vi "LaserCalibration.vi"() -> ()   [LabVIEW 2012]
uses:
  <vilib>/Utility/file.llb/Read From Spreadsheet File (DBL).vi
  <vilib>/Utility/file.llb/Write To Spreadsheet File (DBL).vi
  <vilib>/Analysis/NI_AALPro.lvlib
panel:
  out "slope 2":dbl
  out "slope":dbl
  out "Power vs. Voltage":cluster{"all rows":dbl[], "all rows":dbl[]}[](graph)
  out "Output Voltage":dbl(knob) scale=0.0..5.0
  in  "Steps":i32
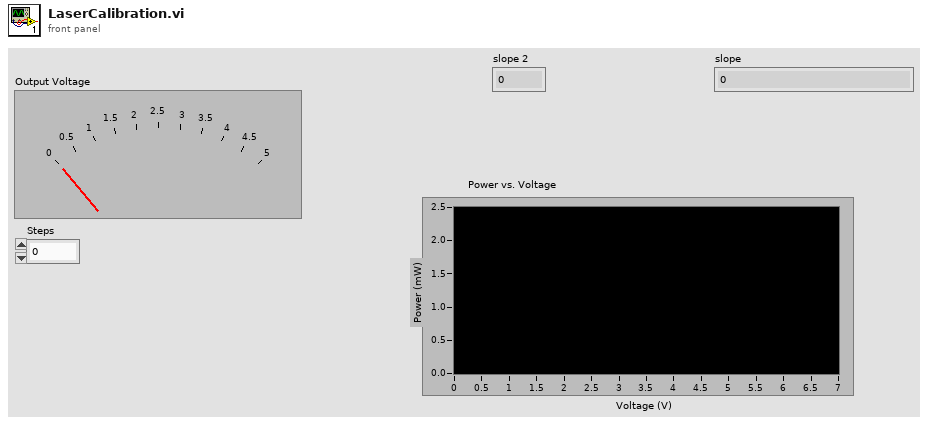
[diagram p1: front panel]
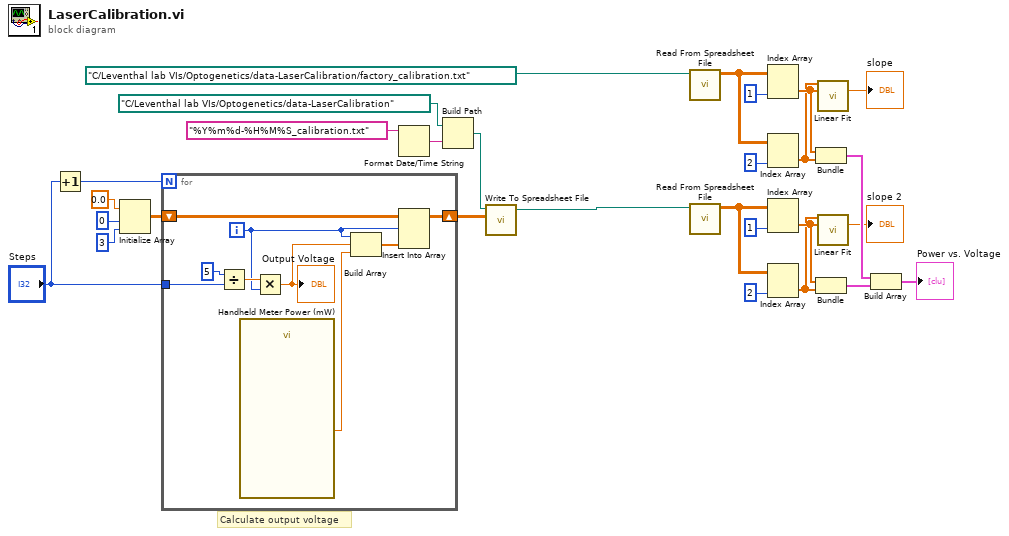
[diagram p0: block diagram]
diagram:
  # "Calculate output voltage"
  n1 = Increment(x="Steps") -> (x+1=w17:i32)
  n2 = Initialize Array(0.0 ("element"), 0 ("dimension size"), 3 ("dimension size")) -> (w15:dbl[][])
  n3 = for {
    N: w17 -> [_]
    shift-right: [w30] -> w11
    shift-left: w15 -> [w31]
    tunnel: "Steps" -> [w37]
    i -> [w32]
    n4 = Divide(x=5, y=w37) -> (x/y=w36:dbl)
    n5 = call "Handheld Meter Power (mW)"() -> ("Power (mW)"=w33:dbl)  [unwired: 17 in, 2 out]
    n6 = Multiply(x=w36, y=w32) -> (x*y=w34:dbl)
    "Output Voltage" <- w34
    n7 = Build Array(w32, w34, w33) -> (w29:dbl[])
    n8 = Insert Into Array(array=w31, index (row)=w32, new element=w29) -> (w30:dbl[][])  [unwired: 1 in]
  }
  n9 = Format Date/Time String(time format string (%c)="%Y%m%d-%H%M%S_calibration.txt") -> (date/time string=w19:string)  [unwired: 2 in]
  n10 = Build Path(base path=path "C:/Leventhal lab VIs/Optogenetics/data-LaserCalibration" ("Path"), name or relative path=w19) -> (appended path=w10:path)
  n11 = call-poly <vilib>:"Write To Spreadsheet File.vi"("2D data"=w11, "file path (dialog if empty)"=w10) -> ("new file path (Not A Path if cancelled)"=w7:path)  [unwired: 6 in]
  n12 = call-poly <vilib>:"Read From Spreadsheet File.vi"("file path (dialog if empty)"=path "C:/Leventhal lab VIs/Optogenetics/data-LaserCalibration/factory_calibration.txt") -> ("all rows"=w26:dbl[][])  [unwired: 6 in, 4 out]
  n13 = call-poly <vilib>:"Read From Spreadsheet File.vi"("file path (dialog if empty)"=w7) -> ("all rows"=w8:dbl[][])  [unwired: 6 in, 4 out]
  n14 = Index Array(array=w26, index (col)=1 ("index (row)")) -> (element=w6:dbl[])  [unwired: 1 in]
  n15 = Index Array(array=w26, index (col)=2 ("disabled index (col)")) -> (element=w5:dbl[])  [unwired: 1 in]
  n16 = Index Array(array=w8, index (col)=1 ("index (row)")) -> (element=w3:dbl[])  [unwired: 1 in]
  n17 = Index Array(array=w8, index (col)=2 ("disabled index (col)")) -> (element=w2:dbl[])  [unwired: 1 in]
  n18 = Bundle "Bundle"("all rows"=w6, "all rows"=w5) -> (w21:cluster{"all rows":dbl[], "all rows":dbl[]})  [unwired: 1 in]
  n19 = Bundle "Bundle"("all rows"=w3, "all rows"=w2) -> (w22:cluster{"all rows":dbl[], "all rows":dbl[]})  [unwired: 1 in]
  n20 = call <vilib>:"Linear Fit.vi"("Y"=w5, "X"=w6) -> ("slope"=→"slope":dbl)  [unwired: 9 in, 4 out]
  n21 = call <vilib>:"Linear Fit.vi"("Y"=w2, "X"=w3) -> ("slope"=→"slope 2":dbl)  [unwired: 9 in, 4 out]
  n22 = Build Array(w21, w22) -> (→"Power vs. Voltage":cluster{"all rows":dbl[], "all rows":dbl[]}[])
